vi "ballrackrange2.vi"   [LabVIEW 2016, in "Test2.lvrbt"]
uses:
  Test2.lvrbt
  <vilib>/NXT/Block Support/NXT_InputPort.ctl
  <vilib>/NXT/Hardware/Plugins/Tetrix DC Motor/TetrixDCMotorAddress.ctl
  <vilib>/NXT/NXTIO Xnodes/NXTIONodeSubVIs/TETRIX IO Move DC Motors.vi
  <vilib>/NXT/Dual Mode Library/Waits/Wait_EV3_Ultrasonic_Centimeter_Closer.vi
  <vilib>/NXT/NXTIO Xnodes/NXTIONodeSubVIs/TETRIX IO Stop DC Motors.vi
  <vilib>/NXT/Dual Mode Library/Waits/Wait_Num.vi
  <vilib>/NXT/Dual Mode Library/Waits/Wait_Touch.vi
  <vilib>/NXT/Dual Mode Library/Waits/Wait_EV3_Ultrasonic_Centimeters_Further.vi
  <vilib>/NXT/Subs/LVHSConnector.ctl
  <vilib>/NXT/NXTIO Xnodes/AddressXNode/NXTIOAddress.xnode
  <vilib>/NXT/NXTIO Xnodes/NXTIOXNode/NXTIO.xnode
  <vilib>/NXT/LegoClasses/BrickReference/BrickReference.lvclass
types:
  T1 = typedef "NXT_InputPort.ctl" = u32
  T2 = typedef "TetrixDCMotorAddress.ctl" = i32
  T3 = typedef "LVHSConnector.ctl" = refnum<class "BrickReference.lvclass">
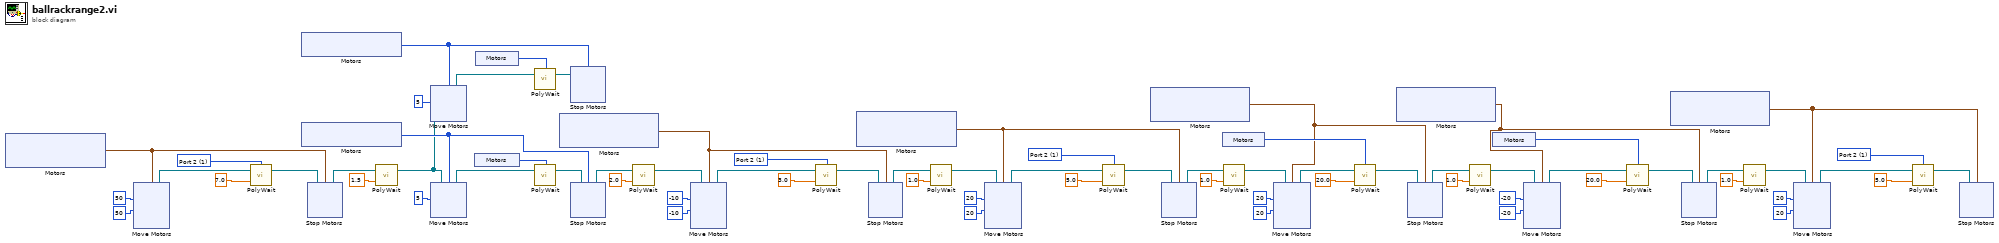
[diagram p0: block diagram]
diagram:
  w4 = T1 1 items=["Port 1", "Port 2", "Port 3", "Port 4"] ("Port (Port 1)")
  w30 = T1 1 items=["Port 1", "Port 2", "Port 3", "Port 4"] ("Port (Port 1)")
  w43 = T1 1 items=["Port 1", "Port 2", "Port 3", "Port 4"] ("Port (Port 1)")
  w51 = T1 1 items=["Port 1", "Port 2", "Port 3", "Port 4"] ("Port (Port 1)")
  n1 = xnode "Motors"() -> ("Motor"=w65:cluster{"TetrixDCMotor":T2, "TetrixDCMotor":T2})
  n2 = xnode "Move Motors"("Power/Speed 2"=i8 50, "Power/Speed 1"=i8 50, "Motors"=w65) -> ("NXT/EV3"=w68:T3)  [unwired: 1 in]
  n3 = call-poly <vilib>:"PolyWait.vi"("Centimeters (40)"=sgl 7.0, "NXT/EV3"=w68, "Port (Port 1)"=w51) -> ("NXT/EV3"=w66:T3)  [unwired: 1 in]
  n4 = xnode "Motors"() -> ("Motor"=w61:T2)
  n5 = xnode "Motors"() -> ("Motor"=w56:T2)
  n6 = xnode "Stop Motors"("Motors"=w65, "NXT/EV3"=w66) -> ("NXT/EV3"=w59:T3)
  n7 = call-poly <vilib>:"PolyWait.vi"("Time (1 sec)"=sgl 1.5, "NXT/EV3"=w59) -> ("NXT/EV3"=w54:T3)  [unwired: 2 in]
  n8 = xnode "Move Motors"("Power/Speed 1"=i8 5, "Motors"=w61, "NXT/EV3"=w54) -> ("NXT/EV3"=w63:T3)
  n9 = xnode "Move Motors"("Power/Speed 1"=i8 5, "Motors"=w56, "NXT/EV3"=w54) -> ("NXT/EV3"=w57:T3)
  n10 = xnode "Motors"() -> ("Sensor"=w53:T1)
  n11 = xnode "Motors"() -> ("Sensor"=w52:T1)
  n12 = call-poly <vilib>:"PolyWait.vi"("NXT/EV3"=w63, "Port (Port 1)"=w52) -> ("NXT/EV3"=w62:T3)  [unwired: 2 in]
  n13 = call-poly <vilib>:"PolyWait.vi"("NXT/EV3"=w57, "Port (Port 1)"=w53) -> ("NXT/EV3"=w55:T3)  [unwired: 2 in]
  n14 = xnode "Motors"() -> ("Motor"=w45:cluster{"TetrixDCMotor":T2, "TetrixDCMotor":T2})
  n15 = xnode "Stop Motors"("Motors"=w61, "NXT/EV3"=w62) -> ()  [unwired: 1 out]
  n16 = xnode "Stop Motors"("Motors"=w56, "NXT/EV3"=w55) -> ("NXT/EV3"=w49:T3)
  n17 = call-poly <vilib>:"PolyWait.vi"("Time (1 sec)"=sgl 2.0, "NXT/EV3"=w49) -> ("NXT/EV3"=w41:T3)  [unwired: 2 in]
  n18 = xnode "Move Motors"("Power/Speed 2"=i8 -10, "Power/Speed 1"=i8 -10, "Motors"=w45, "NXT/EV3"=w41) -> ("NXT/EV3"=w47:T3)
  n19 = call-poly <vilib>:"PolyWait.vi"("Centimeters (50)"=sgl 3.0, "NXT/EV3"=w47, "Port (Port 1)"=w43) -> ("NXT/EV3"=w46:T3)  [unwired: 1 in]
  n20 = xnode "Motors"() -> ("Motor"=w33:cluster{"TetrixDCMotor":T2, "TetrixDCMotor":T2})
  n21 = xnode "Stop Motors"("Motors"=w45, "NXT/EV3"=w46) -> ("NXT/EV3"=w40:T3)
  n22 = call-poly <vilib>:"PolyWait.vi"("Time (1 sec)"=sgl 1.0, "NXT/EV3"=w40) -> ("NXT/EV3"=w1:T3)  [unwired: 2 in]
  n23 = xnode "Move Motors"("Power/Speed 2"=i8 20, "Power/Speed 1"=i8 20, "Motors"=w33, "NXT/EV3"=w1) -> ("NXT/EV3"=w36:T3)
  n24 = call-poly <vilib>:"PolyWait.vi"("Centimeters (50)"=sgl 5.0, "NXT/EV3"=w36, "Port (Port 1)"=w30) -> ("NXT/EV3"=w34:T3)  [unwired: 1 in]
  n25 = xnode "Motors"() -> ("Motor"=w23:cluster{"TetrixDCMotor":T2, "TetrixDCMotor":T2})
  n26 = xnode "Stop Motors"("Motors"=w33, "NXT/EV3"=w34) -> ("NXT/EV3"=w31:T3)
  n27 = xnode "Motors"() -> ("Sensor"=w25:T1)
  n28 = call-poly <vilib>:"PolyWait.vi"("Time (1 sec)"=sgl 1.0, "NXT/EV3"=w31) -> ("NXT/EV3"=w22:T3)  [unwired: 2 in]
  n29 = xnode "Move Motors"("Power/Speed 2"=i8 20, "Power/Speed 1"=i8 20, "Motors"=w23, "NXT/EV3"=w22) -> ("NXT/EV3"=w27:T3)
  n30 = call-poly <vilib>:"PolyWait.vi"("Centimeters (40)"=sgl 20.0, "NXT/EV3"=w27, "Port (Port 1)"=w25) -> ("NXT/EV3"=w24:T3)  [unwired: 1 in]
  n31 = xnode "Motors"() -> ("Motor"=w14:cluster{"TetrixDCMotor":T2, "TetrixDCMotor":T2})
  n32 = xnode "Stop Motors"("Motors"=w23, "NXT/EV3"=w24) -> ("NXT/EV3"=w21:T3)
  n33 = call-poly <vilib>:"PolyWait.vi"("Time (1 sec)"=sgl 1.0, "NXT/EV3"=w21) -> ("NXT/EV3"=w17:T3)  [unwired: 2 in]
  n34 = xnode "Motors"() -> ("Sensor"=w12:T1)
  n35 = xnode "Move Motors"("Power/Speed 2"=i8 -20, "Power/Speed 1"=i8 -20, "Motors"=w14, "NXT/EV3"=w17) -> ("NXT/EV3"=w16:T3)
  n36 = call-poly <vilib>:"PolyWait.vi"("Centimeters (50)"=sgl 20.0, "NXT/EV3"=w16, "Port (Port 1)"=w12) -> ("NXT/EV3"=w15:T3)  [unwired: 1 in]
  n37 = xnode "Motors"() -> ("Motor"=w2:cluster{"TetrixDCMotor":T2, "TetrixDCMotor":T2})
  n38 = xnode "Stop Motors"("Motors"=w14, "NXT/EV3"=w15) -> ("NXT/EV3"=w10:T3)
  n39 = call-poly <vilib>:"PolyWait.vi"("Time (1 sec)"=sgl 1.0, "NXT/EV3"=w10) -> ("NXT/EV3"=w7:T3)  [unwired: 2 in]
  n40 = xnode "Move Motors"("Power/Speed 2"=i8 20, "Power/Speed 1"=i8 20, "Motors"=w2, "NXT/EV3"=w7) -> ("NXT/EV3"=w6:T3)
  n41 = call-poly <vilib>:"PolyWait.vi"("Centimeters (50)"=sgl 5.0, "NXT/EV3"=w6, "Port (Port 1)"=w4) -> ("NXT/EV3"=w3:T3)  [unwired: 1 in]
  n42 = xnode "Stop Motors"("Motors"=w2, "NXT/EV3"=w3) -> ()  [unwired: 1 out]
